vi "PSCHN_Temp Variable.vi"() -> (2 "TempVariable":T3)   [LabVIEW 2016]
uses:
  Controls/PSCHN_Card Para.ctl
  Controls/PSCHN_Channel Para.ctl
  C:/Program Files/National Instruments/LabVIEW 2016/user.lib/HBM.QuantumX/HBM.QuantumX.dll
  Program Files/National Instruments/LabVIEW 2016/user.lib/HBM.QuantumX/HBM.QuantumX.dll
panel:
  # "————————————————\nYou could add your temporary variables\nhere.\nThis Control should be saved as a\nvi in your project folder,The proposed vi's block diagram is shown in the picture\n\n\n\n\n\n\n\n————————————————"
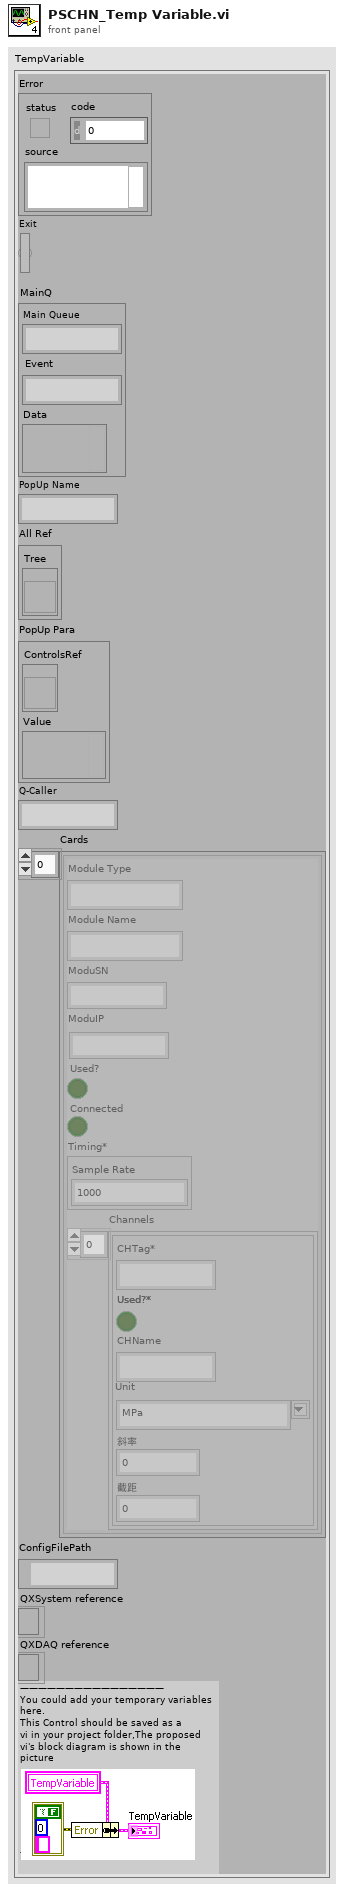
[diagram p1: front panel]
types:
  T1 = typedef "PSCHN_Card Para.ctl" = cluster{"Module Type":string, "Module Name":string, "ModuSN":string, "ModuIP":string, "Used?":bool, "Connected":bool, "Timing*":cluster{"Sample Rate":dbl}, "Channels":T2[]}
  T2 = typedef "PSCHN_Channel Para.ctl" = cluster{"CHTag*":string, "Used?*":bool, "CHName":string, "Unit":string, "斜率":dbl, "截距":dbl}
  T3 = cluster{"Error":errorcluster, "Exit":bool, "MainQ":cluster{"Main Queue":string, "Event":string, "Data":variant}, "PopUp Name":string, "All Ref":cluster{"Tree":refnum<vi>}, "PopUp Para":cluster{"ControlsRef":refnum<vi>, "Value":variant}, "Q-Caller":string, "Cards":T1[], "ConfigFilePath":path, "QXSystem reference":refnum<k24>, "QXDAQ reference":refnum<k24>}
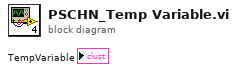
[diagram p0: block diagram]
diagram:
